vi "Custom VISA Selector Demo.vi"() -> ()   [LabVIEW 2020, in "Get COM Descriptor.lvlib"]
doc: "Simple demo app using custom VISA enumeration with COM port names accompanied by their descriptors. It can be used to replace VISA address resource.\n\nDetails: https://github.com/smaslan/get-com-descriptor"
uses:
  Get COM Descriptor.lvlib
  Custom VISA Filters.ctl
panel:
  out "Selected VISA address":refnum<visa-resource-name>
  in  "Interface filter":T1={"GPIB"=TRUE, "Serial"=TRUE, "TCP"=TRUE, "USB"=TRUE}
  in  "Custom VISA selector":u16(ring) items=["TCPIP0::169.254.83.145::inst0::INSTR", "TCPIP0::169.254.143.207::inst0::INSTR", "-", "Refresh"]
  in  "btn exit":bool
  # "Simple demo that replaces LV VISA Address Resource control by custom VISA Ring control. It will display COM port names along with their user descriptor strings obtained using using the get_com_descriptor.dll library. E.g.:\nCOM5: Multiplexer V1.0 (FT232 bridge)\nCOM7: Ambient monitor (CP2102N bridge)"
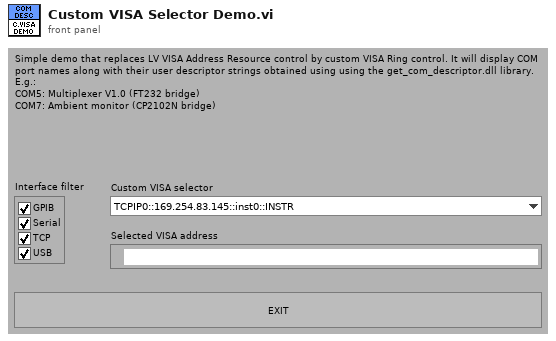
[diagram p1: front panel]
types:
  T1 = typedef "Get COM Descriptor.lvlib/Custom VISA Filters.ctl" = cluster{"GPIB":bool, "Serial":bool, "TCP":bool, "USB":bool}
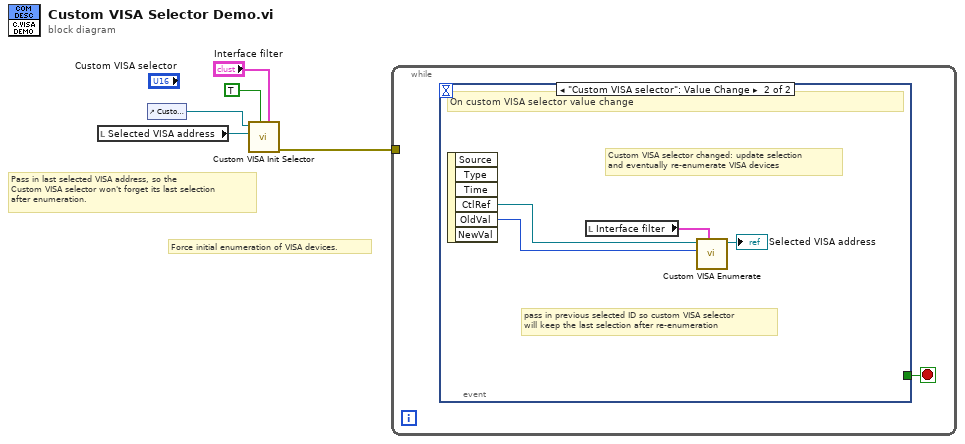
[diagram p0: block diagram]
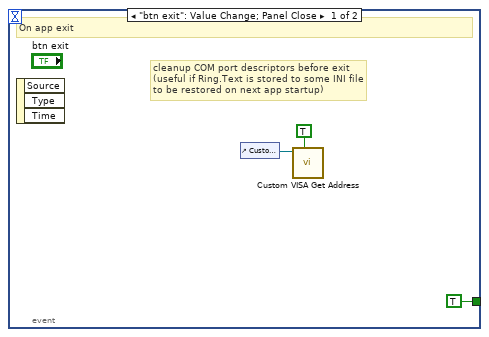
[diagram p2: hidden frame]
diagram:
  # "Pass in last selected VISA address, so the \nCustom VISA selector won't forget its last selection\nafter enumeration."
  # "Force initial enumeration of VISA devices."
  n1 = local read "Selected VISA address"() -> (w5:refnum<visa-resource-name>)
  n2 = control-ref of="Custom VISA selector"() -> (w1:refnum<vi>)
  n3 = call "Custom VISA Init Selector.vi"("Interface filter (all)"="Interface filter", "Initial enumerate? (False)"=TRUE, "VISA address (Empty)"=w5, "VISA menu ref"=w1) -> ("error out"=w2:errorcluster)  [unwired: 7 in]
  n4 = while {
    tunnel: w2 -> [_]
    stop <- w6 stop-if-true
    n5 = event shown="[1] \"Custom VISA selector\": Value Change" {
      selector: _ -> [_ _]
      dyn-events: _ -> [_ _]
      timeout: _ -> [_ _]
      tunnel: [TRUE _] -> w6
      event "btn exit": Value Change; Panel Close {
        # "cleanup COM port descriptors before exit\n(useful if Ring.Text is stored to some INI file\nto be restored on next app startup)"
        # "On app exit"
        n6 = event-data() -> ()  [unwired: 1 in, 3 out]
        n7 = control-ref of="Custom VISA selector"() -> (w7:refnum<vi>)
        n8 = call "Custom VISA Get Address.vi"("Remove COM port descriptor from Ring permanently? (False)"=TRUE, "VISA menu ref"=w7) -> ()  [unwired: 8 in, 2 out]
      }
      event "Custom VISA selector": Value Change {
        # "pass in previous selected ID so custom VISA selector\nwill keep the last selection after re-enumeration"
        # "Custom VISA selector changed: update selection\nand eventually re-enumerate VISA devices"
        # "On custom VISA selector value change"
        n9 = event-data() -> ("CtlRef"=w11:refnum<vi>, "OldVal"=w10:u16)  [unwired: 1 in, 4 out]
        n10 = local read "Interface filter"() -> (w13:T1)
        n11 = call "Custom VISA Enumerate.vi"("Interface filter (all)"=w13, "Last VISA selector Value (none)"=w10, "VISA menu ref"=w11) -> ("Selected VISA address"=→"Selected VISA address":refnum<visa-resource-name>)  [unwired: 6 in, 2 out]
      }
    }
  }
